vi "Quiz #1.vi"() -> ()   [LabVIEW 2019]
panel:
  out "String":string
  out "x+y":dbl
  out "subarray":dbl[](array[numeric])
  out "ANGULOS":dbl[](array[numeric])
  in  "COORDENADA Y":dbl
  in  "COORDENADA X":dbl
  out "VECTORES B":dbl[](array[numeric])
  out "VECTORES A":dbl[](array[numeric])
  in  "Y":dbl[](array[numeric])
  in  "X":dbl[](array[numeric])
  out "PUNTOS COORDENADOS":cluster{"X":dbl[], "Y":dbl[]}(graph)
  out "B2":dbl
  out "B1":dbl
  out "A2":dbl
  out "A1":dbl
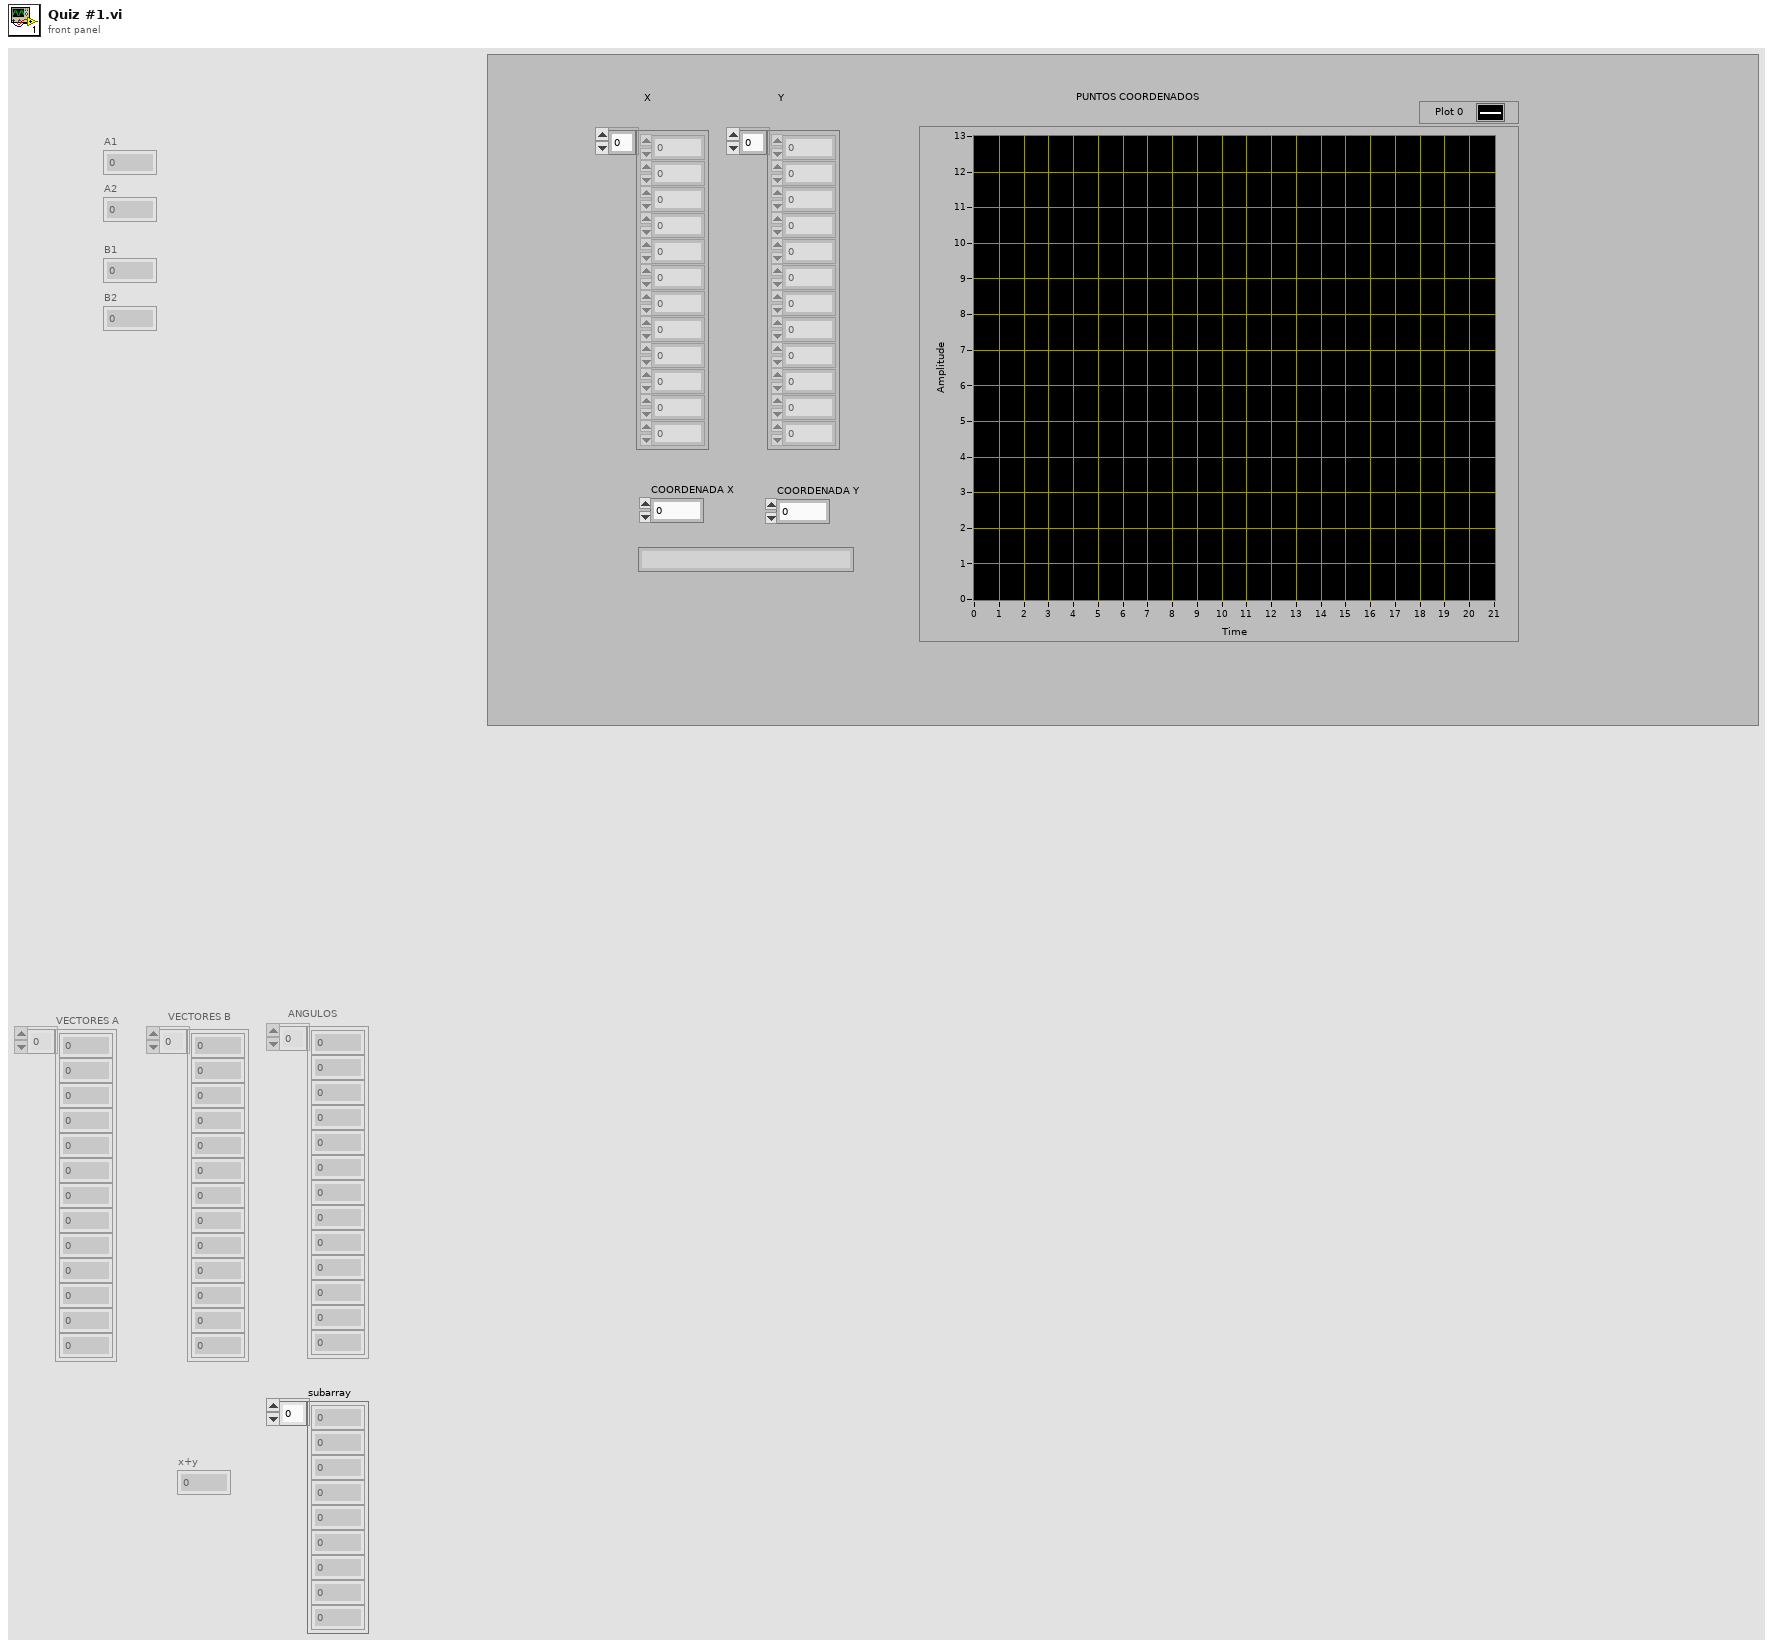
[diagram p1: front panel]
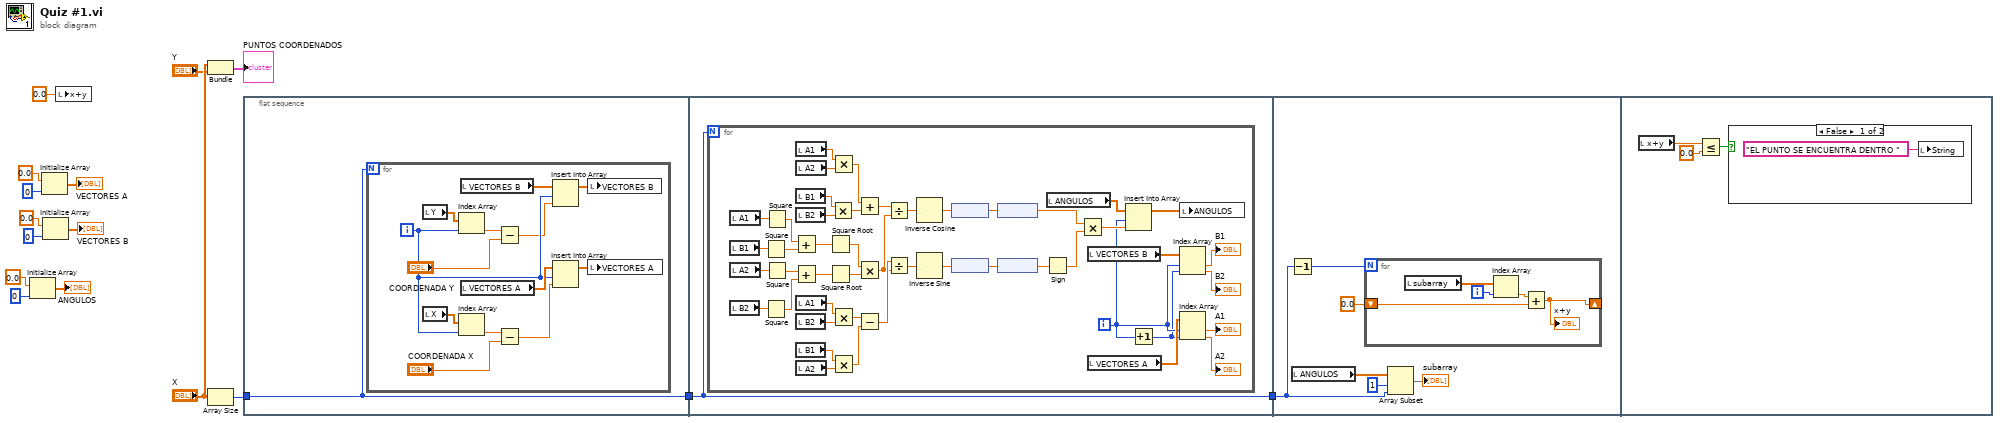
[diagram p0: block diagram]
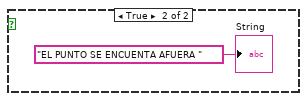
[diagram p2: hidden frame]
diagram:
  n1 = Initialize Array(0.0 ("element"), 0 ("dimension size")) -> (→"ANGULOS":dbl[])
  n2 = Initialize Array(0.0 ("element"), 0 ("dimension size")) -> (→"VECTORES A":dbl[])
  n3 = Initialize Array(0.0 ("element"), 0 ("dimension size")) -> (→"VECTORES B":dbl[])
  n4 = local write "x+y"(0.0 ("x+y")) -> ()
  n5 = Bundle("X"="X", "Y"="Y") -> (→"PUNTOS COORDENADOS":cluster{"X":dbl[], "Y":dbl[]})  [unwired: 1 in]
  n6 = Array Size(array="X") -> (size(s)=w4:i32)
  n7 = flat-sequence {
    tunnel: w4 -> [w17]
    tunnel: [w17] -> w3
    tunnel: w3 -> [w31]
    tunnel: [w31] -> w2
    tunnel: w2 -> [w80]
    frame #0 {
      n8 = for {
        N: w17 -> [_]
        i -> [w21]
        n9 = local read "Y"() -> (w30:dbl[])
        n10 = local read "X"() -> (w29:dbl[])
        n11 = Index Array(array=w30, index=w21) -> (element=w26:dbl)
        n12 = Index Array(array=w29, index=w21) -> (element=w28:dbl)
        n13 = local read "VECTORES B"() -> (w18:dbl[])
        n14 = local read "VECTORES A"() -> (w22:dbl[])
        n15 = Subtract(x=w26, y="COORDENADA Y") -> (x-y=w20:dbl)
        n16 = Subtract(x=w28, y="COORDENADA X") -> (x-y=w24:dbl)
        n17 = Insert Into Array(array=w18, index=w21, new element=w20) -> (w19:dbl[])
        n18 = Insert Into Array(array=w22, index=w21, new element=w24) -> (w23:dbl[])
        n19 = local write "VECTORES B"(w19) -> ()
        n20 = local write "VECTORES A"(w23) -> ()
      }
    }
    frame #1 {
      n21 = for {
        N: w31 -> [_]
        i -> [w47]
        n22 = local read "A1"() -> (w78:dbl)
        n23 = local read "B1"() -> (w76:dbl)
        n24 = local read "A2"() -> (w74:dbl)
        n25 = local read "B2"() -> (w73:dbl)
        n26 = Square(x=w76) -> (x^2=w77:dbl)
        n27 = Square(x=w73) -> (x^2=w72:dbl)
        n28 = Square(x=w78) -> (x^2=w75:dbl)
        n29 = Square(x=w74) -> (x^2=w71:dbl)
        n30 = Add(x=w75, y=w77) -> (x+y=w70:dbl)
        n31 = Add(x=w71, y=w72) -> (x+y=w67:dbl)
        n32 = local read "A1"() -> (w38:dbl)
        n33 = local read "A2"() -> (w39:dbl)
        n34 = local read "B1"() -> (w40:dbl)
        n35 = local read "B2"() -> (w41:dbl)
        n36 = local read "A1"() -> (w66:dbl)
        n37 = local read "B2"() -> (w65:dbl)
        n38 = local read "B1"() -> (w64:dbl)
        n39 = local read "A2"() -> (w63:dbl)
        n40 = Square Root(x=w70) -> (sqrt(x)=w69:dbl)
        n41 = Square Root(x=w67) -> (sqrt(x)=w68:dbl)
        n42 = Multiply(x=w40, y=w41) -> (x*y=w36:dbl)
        n43 = Multiply(x=w38, y=w39) -> (x*y=w37:dbl)
        n44 = Multiply(x=w66, y=w65) -> (x*y=w62:dbl)
        n45 = Multiply(x=w64, y=w63) -> (x*y=w61:dbl)
        n46 = Add(x=w37, y=w36) -> (x+y=w35:dbl)
        n47 = Multiply(x=w69, y=w68) -> (x*y=w34:dbl)
        n48 = Subtract(x=w62, y=w61) -> (x-y=w60:dbl)
        n49 = Divide(x=w35, y=w34) -> (x/y=w53:dbl)
        n50 = Divide(x=w60, y=w34) -> (x/y=w33:dbl)
        n51 = Inverse Cosine(1:w53) -> (0:w50:dbl)
        n52 = Inverse Sine(1:w33) -> (0:w32:dbl)
        n53 = node(w50) -> (w51:dbl[unit])
        n54 = node(w32) -> (w59:dbl[unit])
        n55 = node(w51) -> (w52:dbl)
        n56 = node(w59) -> (w58:dbl)
        n57 = Sign(1:w58) -> (0:w57:dbl)
        n58 = local read "ANGULOS"() -> (w54:dbl[])
        n59 = Multiply(x=w52, y=w57) -> (x*y=w56:dbl)
        n60 = local read "VECTORES B"() -> (w48:dbl[])
        n61 = local read "VECTORES A"() -> (w49:dbl[])
        n62 = Insert Into Array(array=w54, index=w47, new element=w56) -> (w55:dbl[])
        n63 = Increment(x=w47) -> (x+1=w46:i32)
        n64 = local write "ANGULOS"(w55) -> ()
        n65 = Index Array(array=w48, index #1=w47, index #2=w46) -> (element #1=→"B1":dbl, element #2=→"B2":dbl)
        n66 = Index Array(array=w49, index #1=w47, index #2=w46) -> (element #1=→"A1":dbl, element #2=→"A2":dbl)
      }
    }
    frame #2 {
      n67 = Decrement(x=w80) -> (x-1=w81:i32)
      n68 = local read "ANGULOS"() -> (w84:dbl[])
      n69 = for {
        N: w81 -> [_]
        shift-right: [w86] -> _
        shift-left: 0.0 -> [w85]
        i -> [w88]
        n70 = local read "subarray"() -> (w89:dbl[])
        n71 = Index Array(array=w89, index=w88) -> (element=w87:dbl)
        n72 = Add(x=w87, y=w85) -> (x+y=w86:dbl)
        "x+y" <- w86
      }
      n73 = Array Subset(array=w84, index=1, length=w80) -> (→"subarray":dbl[])
    }
    frame #3 {
      n74 = local read "x+y"() -> (w92:dbl)
      n75 = Less Or Equal?(x=w92, y=0.0) -> (x <= y?=w90:bool)
      n76 = case shown="False" w90 {
        frame False {
          n77 = local write "String"("EL PUNTO SE ENCUENTRA DENTRO " ("String")) -> ()
        }
        frame True {
          "String" <- "EL PUNTO SE ENCUENTA AFUERA "
        }
      }
    }
  }
